vi "Periodic Tasks.vi"(8 "error in":errorcluster) -> ()   [LabVIEW 2013]
doc: "This VI runs in parallel to other tasks. It can contain as many user-defined periodic loops as you need. These can carry out PID or other sorts of timed response."
uses:
  <vilib>/Rock Robotics/SystemInterfaces/Utilities/FPGA_UtilitiesLED Source.ctl
  <vilib>/Rock Robotics/SystemInterfaces/Utilities/FPGA_UtilitiesLED State.ctl
  <vilib>/Rock Robotics/WPI/Joystick/WPI_JoystickGetSetRefNum.vi
  Robot Global Data.vi
  <vilib>/addons/control/pid/pid.llb/PID (DBL).vi
  <vilib>/addons/control/pid/NI_PID_pid.lvlib
panel:
  out "Voltage 2":dbl
  out "Voltage":dbl
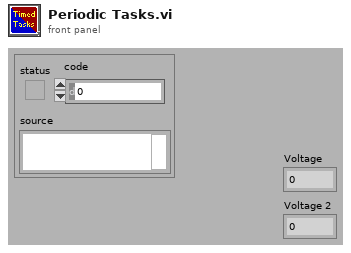
[diagram p1: front panel]
types:
  T1 = typedef "WPI_EncoderDevRef.ctl" = cluster{"DevStatus":errorcluster, "EncoderIndex":T2, "CounterIndex":T3, "DistancePerCount":dbl, "Decoding Type":T4}
  T2 = typedef "FPGA_EncoderIdx.ctl" = enum8{"Enc 0", "Enc 1", "Enc 2", "Enc 3", "Invalid"}
  T3 = typedef "FPGA_CounterCtrSystemIndex.ctl" = enum8{"Ctr 0", "Ctr 1", "Ctr 2", "Ctr 3", "Ctr 4", "Ctr 5", "Ctr 6", "Ctr 7", "Invalid"}
  T4 = typedef "WPI_EncoderType.ctl" = enum16{"1x", "2x", "4x"}
  T5 = typedef "WPI_MotorControlDeviceRef.ctl" = cluster{"DeviceStatus":errorcluster, "Type":enum16{"PWM", "CAN"}, "PWM":cluster{"Digital Module":T6, "PWM Channel":T7, "DeadBand":T8}, "CAN":cluster{"Device Number":u8, "Control Mode":T9, "Semaphore":T10, "Max Vout":dbl}, "Invert":bool, "TransformRef":T11, "InvTransformRef":T11}
  T6 = typedef "FPGA_TypedefDigitalModule.ctl" = enum16{"Digital Module 1", "Digital Module 2"}
  T7 = typedef "FPGA_DIOPWMChannel.ctl" = enum8{"PWM 1", "PWM 2", "PWM 3", "PWM 4", "PWM 5", "PWM 6", "PWM 7", "PWM 8", "PWM 9", "PWM 10", "Invalid"}
  T8 = typedef "WPI_PWMDeadband.ctl" = cluster{"Name":string, "maxPositivePwm":i32, "minPositivePwm":i32, "centerPwm":i32, "maxNegativePwm":i32, "minNegativePwm":i32, "angularRange":u16}
  T9 = typedef "WPI_CANJaguar_ControlMode.ctl" = enum8{"Percent VBus", "Current", "Speed", "Position", "Voltage"}
  T10 = typedef "Semaphore RefNum" = refnum<k1>
  T11 = typedef "WPI_PWMTransform_ConPane.ctl" = refnum<vi>
  T12 = typedef "WPI_AnalogChannelDevRef.ctl" = cluster{"DevStatus":errorcluster, "Analog Module":T13, "Analog Channel":T14}
  T13 = typedef "FPGA_TypedefAnalogModule.ctl" = enum16{"Analog Module 1", "Analog Module 2"}
  T14 = typedef "FPGA_AIChannel.ctl" = enum8{"AI 1", "AI 2", "AI 3", "AI 4", "AI 5", "AI 6", "AI 7", "AI 8", "Invalid"}
  T15 = typedef "WPI_JoystickDevRef.ctl" = cluster{"Device":T16}
  T16 = typedef "WPI_JoystickDeviceEnum.ctl" = enum16{"USB 1", "USB 2", "USB 3", "USB 4", "Kinect 1", "Kinect 2"}
  T17 = cluster{"proportional gain (Kc)":dbl, "integral time (Ti, min)":dbl, "derivative time (Td, min)":dbl}
  T18 = enum16{"Default", "Set", "Pickup", "Place", "KickerUp", "Rest", "Kick", "Rest2", "Up", "End"}
  T19 = enum16{"Default", "Set", "Pickup", "Place", "KickerUp", "Rest", "Kick", "End"}
  T20 = cluster{dbl, "integral time (Ti, min)":dbl, "derivative time (Td, min)":dbl}
  T21 = typedef "WPI_JoystickButtonState.ctl" = cluster{"Button 1":bool, "Button 2":bool, "Button 3":bool, "Button 4":bool, "Button 5":bool, "Button 6":bool, "Button 7":bool, "Button 8":bool, "Button 9":bool, "Button 10":bool, "Button 11":bool, "Button 12":bool}
  T22 = cluster{"axis 1 (x)":dbl, "axis 2 (y)":dbl, "axis 3 (throttle)":dbl, "axis 4":dbl, "axis 5":dbl, "axis 6":dbl}
  T23 = typedef "FPGA_UtilitiesLED State.ctl" = enum16{"Off", "On", "Toggle"}
  T24 = typedef "FPGA_UtilitiesLED Source.ctl" = enum16{"User LED", "FPGA LED"}
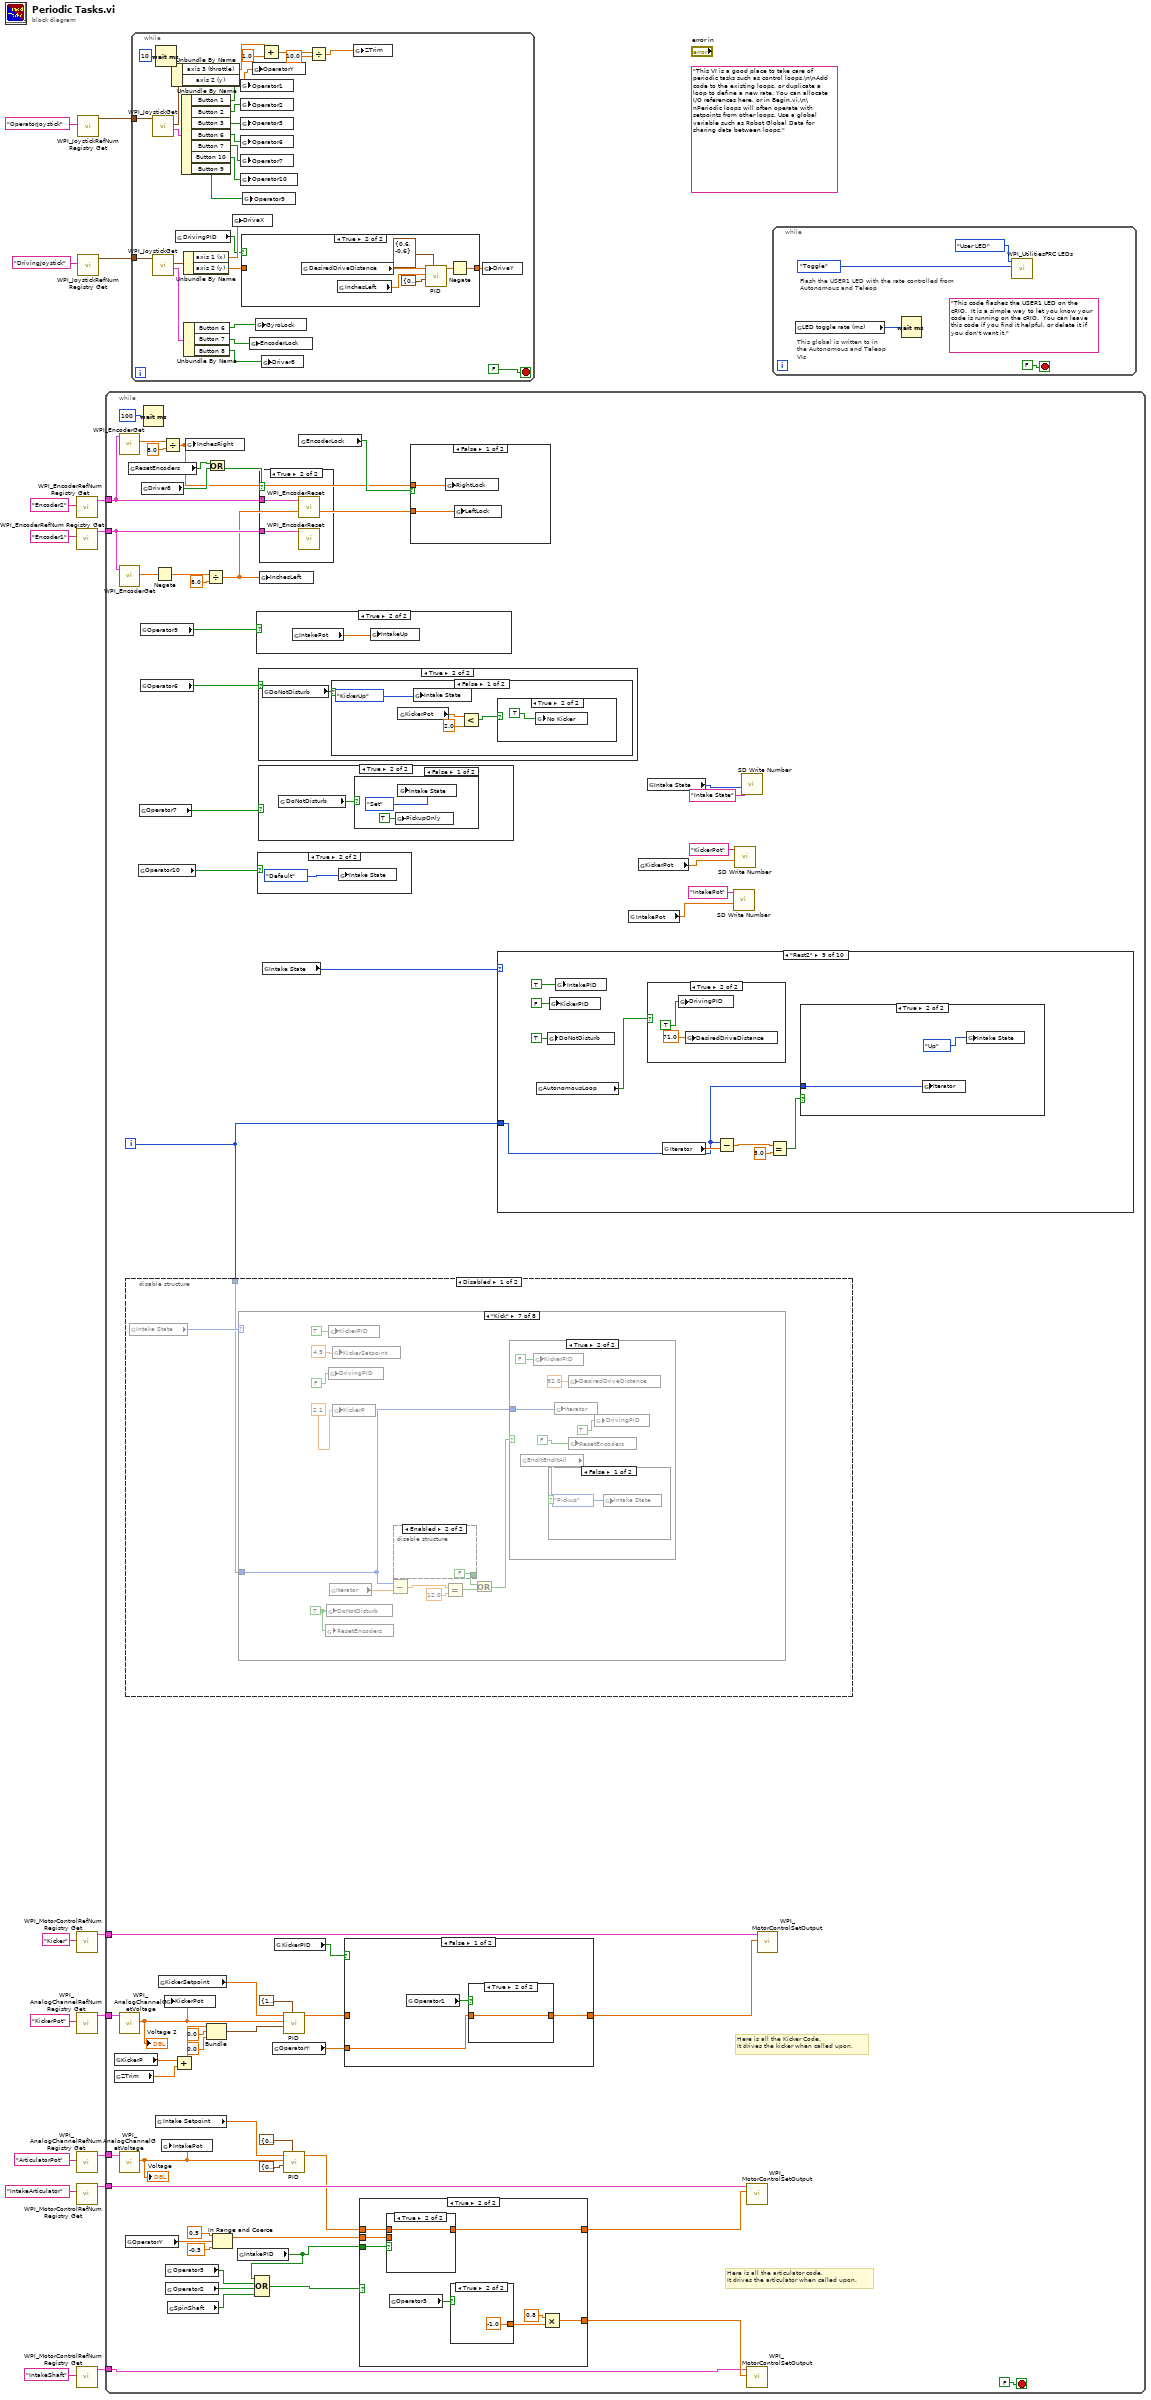
[diagram p0: block diagram]
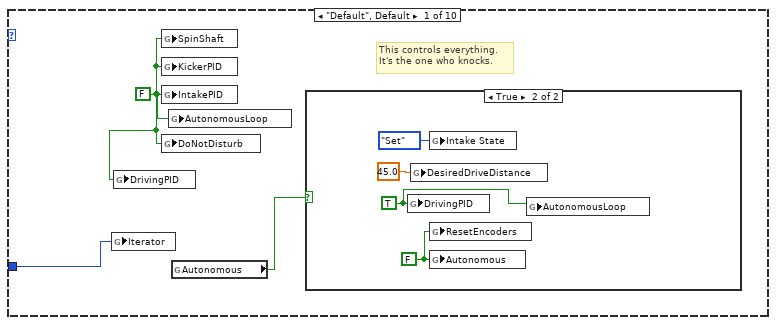
[diagram p2: hidden frame]
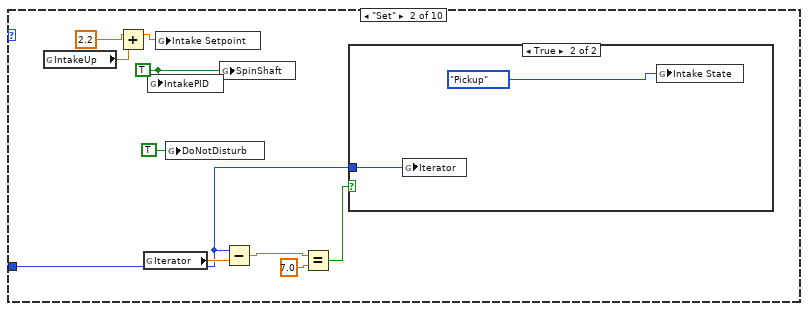
[diagram p4: hidden frame]
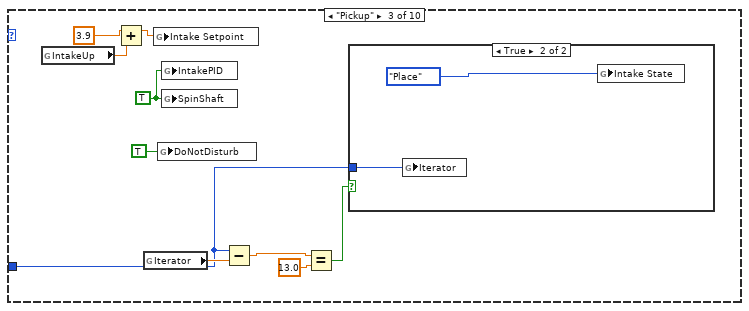
[diagram p6: hidden frame]
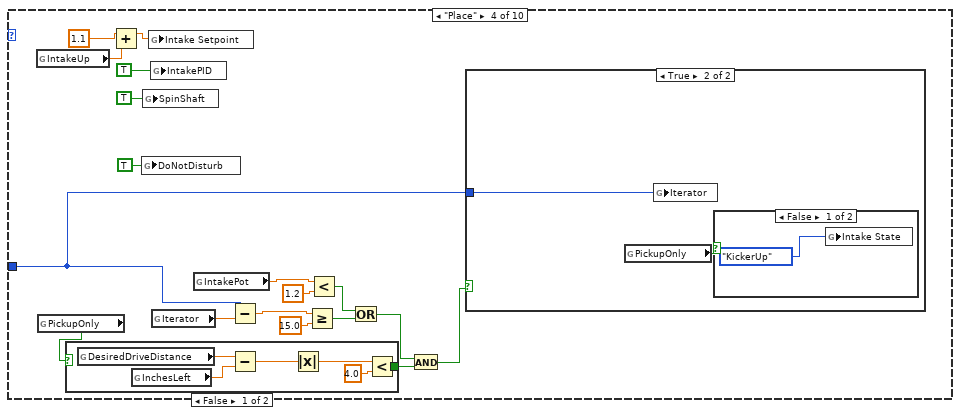
[diagram p8: hidden frame]
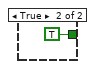
[diagram p9: hidden frame]
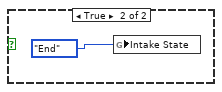
[diagram p11: hidden frame]
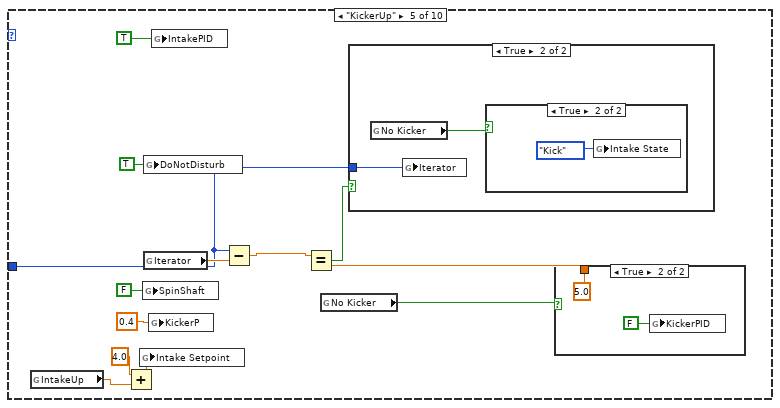
[diagram p12: hidden frame]
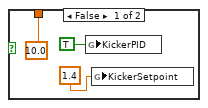
[diagram p13: hidden frame]
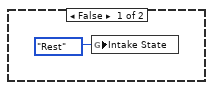
[diagram p15: hidden frame]
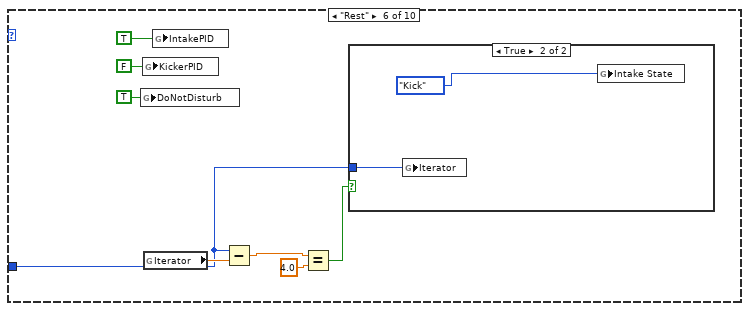
[diagram p16: hidden frame]
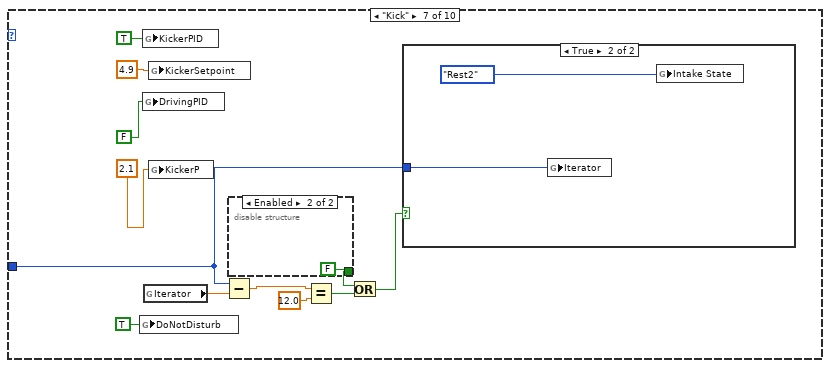
[diagram p18: hidden frame]
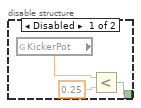
[diagram p19: hidden frame]
diagram:
  (unwired) "This VI is a good place to take care of periodic tasks such as control loops.\n\nAdd code to the existing loops, or duplicate a loop to define a new rate. You can allocate I/O references here, or in Begin.vi.\n\nPeriodic loops will often operate with setpoints from other loops. Use a global variable such as Robot Global Data for sharing data between loops."
  n1 = call <vilib>:"WPI_EncoderRefNum Registry Get.vi"("refnum name"="Encoder2") -> ("EncoderDevRef"=w12:T1)  [unwired: 9 in, 1 out]
  n2 = call <vilib>:"WPI_EncoderRefNum Registry Get.vi"("refnum name"="Encoder1") -> ("EncoderDevRef"=w13:T1)  [unwired: 9 in, 1 out]
  n3 = call <vilib>:"WPI_MotorControlRefNum Registry Get.vi"("refnum name"="Kicker") -> ("MotorControlDevRef"=w7:T5)  [unwired: 9 in, 1 out]
  n4 = call <vilib>:"WPI_AnalogChannelRefNum Registry Get.vi"("refnum name"="KickerPot") -> ("AIDeviceRef"=w4:T12)  [unwired: 9 in, 1 out]
  n5 = call <vilib>:"WPI_AnalogChannelRefNum Registry Get.vi"("refnum name"="ArticulatorPot") -> ("AIDeviceRef"=w3:T12)  [unwired: 9 in, 1 out]
  n6 = call <vilib>:"WPI_MotorControlRefNum Registry Get.vi"("refnum name"="IntakeArticulator") -> ("MotorControlDevRef"=w17:T5)  [unwired: 9 in, 1 out]
  n7 = call <vilib>:"WPI_MotorControlRefNum Registry Get.vi"("refnum name"="IntakeShaft") -> ("MotorControlDevRef"=w14:T5)  [unwired: 9 in, 1 out]
  n8 = call <vilib>:"WPI_JoystickRefNum Registry Get.vi"("refnum name"="OperatorJoystick") -> ("JoystickDevRef"=w1:T15)  [unwired: 9 in, 1 out]
  n9 = call <vilib>:"WPI_JoystickRefNum Registry Get.vi"("refnum name"="DrivingJoystick") -> ("JoystickDevRef"=w9:T15)  [unwired: 9 in, 1 out]
  n10 = while {
    tunnel: w17 -> [w77]
    tunnel: w14 -> [w75]
    tunnel: w13 -> [w59]
    tunnel: w12 -> [w62]
    tunnel: w7 -> [w70]
    tunnel: w4 -> [w69]
    tunnel: w3 -> [w68]
    i -> [w28]
    stop <- FALSE stop-if-true
    # "Here is all the articulator code. \nIt drives the articulator when called upon."
    # "Here is all the Kicker Code. \nIt drives the kicker when called upon."
    n11 = global read "Robot Global Data.vi" "KickerP"() -> (w50:dbl)
    n12 = global read "Robot Global Data.vi" "ZTrim"() -> (w32:dbl)
    n13 = call <vilib>:"WPI_EncoderGet.vi"("EncoderDevRef"=w62) -> ("Distance"=w73:dbl)  [unwired: 5 in, 5 out]
    n14 = call <vilib>:"WPI_EncoderGet.vi"("EncoderDevRef"=w59) -> ("Distance"=w74:dbl)  [unwired: 5 in, 5 out]
    n15 = call <vilib>:"WPI_AnalogChannelGetVoltage.vi"("AIDeviceRef"=w69) -> ("Voltage"=w41:dbl)  [unwired: 8 in, 2 out]
    "Voltage 2" <- w41
    n16 = call <vilib>:"WPI_AnalogChannelGetVoltage.vi"("AIDeviceRef"=w68) -> ("Voltage"=w40:dbl)  [unwired: 8 in, 2 out]
    "Voltage" <- w40
    n17 = global read "Robot Global Data.vi" "OperatorY"() -> (w46:dbl)
    n18 = disable-structure shown="Disabled" {
      disable-tunnel: w28 -> [w220 _]
      frame Disabled {
        n19 = global read "Robot Global Data.vi" "Intake State"() -> (w221:T18)
        n20 = case shown="\"Kick\"" w221 {
          tunnel: w220 -> [w224 w232 w244 w268 w285 w299 w311 _]
          frame "Default", Default {
            w222 = FALSE ("PID")
            # "This controls everything. \nIt's the one who knocks."
            n21 = global write "Robot Global Data.vi" "Iterator"(w224) -> ()
            n22 = global read "Robot Global Data.vi" "Operator7"() -> (w223:bool)
            n23 = global write "Robot Global Data.vi" "SpinShaft"(w222) -> ()
            n24 = global write "Robot Global Data.vi" "KickerPID"(w222) -> ()
            n25 = global write "Robot Global Data.vi" "IntakePID"(w222) -> ()
            n26 = global write "Robot Global Data.vi" "DoNotDisturb"(w222) -> ()
            n27 = global write "Robot Global Data.vi" "EndItEndItAll"(w222) -> ()
            n28 = case shown="True" w223 {
              frame False {
              }
              frame True {
                w225 = FALSE ("Autonomous")
                n29 = global write "Robot Global Data.vi" "Intake State"(T19."Set" ("Intake State")) -> ()
                n30 = global write "Robot Global Data.vi" "ResetEncoders"(w225) -> ()
                n31 = global write "Robot Global Data.vi" "Autonomous"(w225) -> ()
              }
            }
          }
          frame "Set" {
            w231 = TRUE ("PID")
            n32 = global read "Robot Global Data.vi" "IntakeUp"() -> (w229:dbl)
            n33 = Add(x=1.1 ("Intake Setpoint"), y=w229) -> (x+y=w228:dbl)
            n34 = global read "Robot Global Data.vi" "Iterator"() -> (w236:dbl)
            n35 = global write "Robot Global Data.vi" "IntakePID"(w231) -> ()
            n36 = global write "Robot Global Data.vi" "Intake Setpoint"(w228) -> ()
            n37 = global write "Robot Global Data.vi" "DoNotDisturb"(TRUE ("DoNotDisturb")) -> ()
            n38 = global write "Robot Global Data.vi" "SpinShaft"(w231) -> ()
            n39 = Subtract(x=w232, y=w236) -> (x-y=w235:dbl)
            n40 = Equal?(x=w235, y=9.0) -> (x = y?=w233:bool)
            n41 = case shown="True" w233 {
              tunnel: w232 -> [_ w238]
              frame False {
              }
              frame True {
                n42 = global write "Robot Global Data.vi" "Iterator"(w238) -> ()
                n43 = global write "Robot Global Data.vi" "Intake State"(T19."KickerUp" ("Intake State")) -> ()
              }
            }
          }
          frame "Pickup" {
            w243 = TRUE ("PID")
            n44 = global read "Robot Global Data.vi" "InchesRight"() -> (w240:dbl)
            n45 = global read "Robot Global Data.vi" "Iterator"() -> (w248:dbl)
            n46 = global write "Robot Global Data.vi" "DoNotDisturb"(TRUE ("DoNotDisturb")) -> ()
            n47 = Greater?(x=w240, y=24.0) -> (0:w241:bool)
            n48 = global write "Robot Global Data.vi" "IntakePID"(w243) -> ()
            n49 = global write "Robot Global Data.vi" "SpinShaft"(w243) -> ()
            n50 = case shown="False" w241 {
              frame False {
                n51 = global read "Robot Global Data.vi" "IntakeUp"() -> (w249:dbl)
                n52 = Add(x=1.1 ("Intake Setpoint"), y=w249) -> (x+y=w250:dbl)
                n53 = global write "Robot Global Data.vi" "Intake Setpoint"(w250) -> ()
              }
              frame True {
                n54 = global read "Robot Global Data.vi" "IntakeUp"() -> (w252:dbl)
                n55 = Add(x=3.9 ("Intake Setpoint"), y=w252) -> (x+y=w253:dbl)
                n56 = global write "Robot Global Data.vi" "Intake Setpoint"(w253) -> ()
              }
            }
            n57 = Subtract(x=w244, y=w248) -> (x-y=w247:dbl)
            n58 = Equal?(x=w247, y=20.0) -> (x = y?=w245:bool)
            n59 = case shown="False" w245 {
              tunnel: w244 -> [_ w256]
              frame False {
              }
              frame True {
                n60 = global write "Robot Global Data.vi" "Iterator"(w256) -> ()
                n61 = global write "Robot Global Data.vi" "Intake State"(T19."Place" ("Intake State")) -> ()
              }
            }
          }
          frame "Place" {
            w257 = TRUE ("DoNotDisturb")
            n62 = global read "Robot Global Data.vi" "IntakeUp"() -> (w260:dbl)
            n63 = global read "Robot Global Data.vi" "PickupOnly"() -> (w259:bool)
            n64 = case shown="True" w259 {
              tunnel: [w274 TRUE] -> _
              frame False {
                n65 = global read "Robot Global Data.vi" "DesiredDriveDistance"() -> (w278:dbl)
                n66 = global read "Robot Global Data.vi" "InchesRight"() -> (w273:dbl)
                n67 = Subtract(x=w278, y=w273) -> (x-y=w277:dbl)
                n68 = Absolute Value(x=w277) -> (abs(x)=w276:dbl)
                n69 = Less?(x=w276, y=2.0) -> (x < y?=w274:bool)
              }
              frame True {
              }
            }
            n70 = Add(x=1.1 ("Intake Setpoint"), y=w260) -> (x+y=w261:dbl)
            n71 = global write "Robot Global Data.vi" "EndItEndItAll"(w257) -> ()
            n72 = global write "Robot Global Data.vi" "DoNotDisturb"(w257) -> ()
            n73 = global write "Robot Global Data.vi" "SpinShaft"(TRUE ("PID")) -> ()
            n74 = global write "Robot Global Data.vi" "Intake Setpoint"(w261) -> ()
            n75 = global write "Robot Global Data.vi" "IntakePID"(TRUE ("PID")) -> ()
            n76 = global read "Robot Global Data.vi" "Iterator"() -> (w272:dbl)
            n77 = global read "Robot Global Data.vi" "IntakePot"() -> (w263:dbl)
            n78 = Subtract(x=w268, y=w272) -> (x-y=w271:dbl)
            n79 = Equal?(x=w271, y=15.0) -> (x = y?=w269:bool)
            n80 = Less?(x=w263, y=1.4) -> (x < y?=w264:bool)
            n81 = Or(x=w264, y=w269) -> (x .or. y?=w258:bool)
            n82 = case shown="True" w258 {
              tunnel: w268 -> [_ w281]
              frame False {
              }
              frame True {
                n83 = global write "Robot Global Data.vi" "Iterator"(w281) -> ()
                n84 = global write "Robot Global Data.vi" "Intake State"(T19."KickerUp" ("Intake State")) -> ()
              }
            }
          }
          frame "KickerUp" {
            n85 = global read "Robot Global Data.vi" "IntakeUp"() -> (w282:dbl)
            n86 = Add(x=4.0 ("Intake Setpoint"), y=w282) -> (x+y=w283:dbl)
            n87 = global write "Robot Global Data.vi" "Intake Setpoint"(w283) -> ()
            n88 = global write "Robot Global Data.vi" "KickerPID"(TRUE ("PID")) -> ()
            n89 = global write "Robot Global Data.vi" "SpinShaft"(FALSE ("PID")) -> ()
            n90 = global write "Robot Global Data.vi" "DoNotDisturb"(TRUE ("DoNotDisturb")) -> ()
            n91 = global read "Robot Global Data.vi" "Iterator"() -> (w289:dbl)
            n92 = global write "Robot Global Data.vi" "KickerSetpoint"(1.4 ("KickerSetpoint")) -> ()
            n93 = global write "Robot Global Data.vi" "KickerP"(0.4 ("KickerP")) -> ()
            n94 = global write "Robot Global Data.vi" "IntakePID"(TRUE ("PID")) -> ()
            n95 = Subtract(x=w285, y=w289) -> (x-y=w288:dbl)
            n96 = Equal?(x=w288, y=10.0) -> (x = y?=w286:bool)
            n97 = case shown="True" w286 {
              tunnel: w285 -> [_ w297]
              frame False {
              }
              frame True {
                n98 = global write "Robot Global Data.vi" "Iterator"(w297) -> ()
                n99 = global write "Robot Global Data.vi" "Intake State"(T19."Rest" ("Intake State")) -> ()
              }
            }
          }
          frame "Rest" {
            n100 = global write "Robot Global Data.vi" "DoNotDisturb"(TRUE ("DoNotDisturb")) -> ()
            n101 = global write "Robot Global Data.vi" "KickerPID"(FALSE ("PID")) -> ()
            n102 = global read "Robot Global Data.vi" "Iterator"() -> (w303:dbl)
            n103 = global write "Robot Global Data.vi" "IntakePID"(TRUE ("PID")) -> ()
            n104 = Subtract(x=w299, y=w303) -> (x-y=w302:dbl)
            n105 = Equal?(x=w302, y=3.0) -> (x = y?=w300:bool)
            n106 = case shown="True" w300 {
              tunnel: w299 -> [_ w307]
              frame False {
              }
              frame True {
                n107 = global write "Robot Global Data.vi" "Iterator"(w307) -> ()
                n108 = global write "Robot Global Data.vi" "Intake State"(T19."Kick" ("Intake State")) -> ()
              }
            }
          }
          frame "Kick" {
            w308 = TRUE ("DoNotDisturb")
            n109 = global write "Robot Global Data.vi" "ResetEncoders"(w308) -> ()
            n110 = global write "Robot Global Data.vi" "DoNotDisturb"(w308) -> ()
            n111 = global write "Robot Global Data.vi" "KickerPID"(TRUE ("PID")) -> ()
            n112 = global write "Robot Global Data.vi" "DrivingPID"(FALSE ("DrivingPID")) -> ()
            n113 = global read "Robot Global Data.vi" "Iterator"() -> (w314:dbl)
            n114 = global write "Robot Global Data.vi" "KickerSetpoint"(4.9 ("KickerSetpoint")) -> ()
            n115 = global write "Robot Global Data.vi" "KickerP"(2.1 ("KickerP")) -> ()
            n116 = Subtract(x=w311, y=w314) -> (x-y=w313:dbl)
            n117 = disable-structure shown="Enabled" {
              disable-tunnel: [w321 FALSE] -> w316
              frame Disabled {
                n118 = global read "Robot Global Data.vi" "KickerPot"() -> (w320:dbl)
                n119 = Less?(x=w320, y=0.25) -> (x < y?=w321:bool)
              }
              frame Enabled {
              }
            }
            n120 = Equal?(x=w313, y=12.0) -> (x = y?=w309:bool)
            n121 = Or(x=w316, y=w309) -> (x .or. y?=w310:bool)
            n122 = case shown="True" w310 {
              tunnel: w311 -> [_ w329]
              frame False {
              }
              frame True {
                n123 = global read "Robot Global Data.vi" "EndItEndItAll"() -> (w325:bool)
                n124 = global write "Robot Global Data.vi" "KickerPID"(FALSE ("PID")) -> ()
                n125 = case shown="False" w325 {
                  frame False {
                    n126 = global write "Robot Global Data.vi" "Intake State"(T19."Pickup" ("Intake State")) -> ()
                  }
                  frame True {
                    n127 = global write "Robot Global Data.vi" "Intake State"(T19."End" ("Intake State")) -> ()
                  }
                }
                n128 = global write "Robot Global Data.vi" "Iterator"(w329) -> ()
                n129 = global write "Robot Global Data.vi" "DesiredDriveDistance"(92.0 ("DesiredDriveDistance")) -> ()
                n130 = global write "Robot Global Data.vi" "ResetEncoders"(FALSE ("DrivingPID")) -> ()
                n131 = global write "Robot Global Data.vi" "DrivingPID"(TRUE ("DrivingPID")) -> ()
              }
            }
          }
          frame "End" {
            w332 = FALSE ("DoNotDisturb")
            w333 = FALSE ("PID")
            n132 = global write "Robot Global Data.vi" "DoNotDisturb"(w332) -> ()
            n133 = global write "Robot Global Data.vi" "KickerPID"(FALSE ("PID")) -> ()
            n134 = global write "Robot Global Data.vi" "IntakePID"(w333) -> ()
            n135 = global write "Robot Global Data.vi" "DrivingPID"(w333) -> ()
            n136 = global write "Robot Global Data.vi" "Intake State"(T19."Default" ("Intake State")) -> ()
            n137 = global write "Robot Global Data.vi" "PickupOnly"(w332) -> ()
          }
        }
      }
      frame Enabled {
      }
    }
    n138 = global read "Robot Global Data.vi" "ResetEncoders"() -> (w35:bool)
    n139 = global read "Robot Global Data.vi" "Operator10"() -> (w37:bool)
    n140 = global read "Robot Global Data.vi" "Operator7"() -> (w38:bool)
    n141 = global read "Robot Global Data.vi" "Operator9"() -> (w31:bool)
    n142 = global read "Robot Global Data.vi" "Operator6"() -> (w39:bool)
    n143 = global read "Robot Global Data.vi" "Driver8"() -> (w34:bool)
    n144 = Wait (ms)(milliseconds to wait=u32 100) -> ()  [unwired: 1 out]
    n145 = Negate(x=w74) -> (-x=w58:dbl)
    n146 = global read "Robot Global Data.vi" "Intake Setpoint"() -> (w63:dbl)
    n147 = global read "Robot Global Data.vi" "KickerSetpoint"() -> (w49:dbl)
    n148 = global write "Robot Global Data.vi" "IntakePot"(w40) -> ()
    n149 = Divide(x=w73, y=8.0) -> (x/y=w19:dbl)
    n150 = global write "Robot Global Data.vi" "KickerPot"(w41) -> ()
    n151 = global read "Robot Global Data.vi" "Operator3"() -> (w43:bool)
    n152 = global read "Robot Global Data.vi" "Operator2"() -> (w42:bool)
    n153 = global read "Robot Global Data.vi" "SpinShaft"() -> (w54:bool)
    n154 = Add(x=w50, y=w32) -> (x+y=w33:dbl)
    n155 = global write "Robot Global Data.vi" "InchesRight"(w19) -> ()
    n156 = Divide(x=w58, y=8.0) -> (x/y=w20:dbl)
    n157 = Bundle(w33, "integral time (Ti, min)"=0.0, "derivative time (Td, min)"=0.0) -> (w53:T20)  [unwired: 1 in]
    n158 = Or(x=w35, y=w34) -> (x .or. y?=w36:bool)
    n159 = In Range and Coerce(upper limit=0.5, x=w46, lower limit=-0.5) -> (coerced(x)=w60:dbl)  [unwired: 1 out]
    n160 = global read "Robot Global Data.vi" "IntakePID"() -> (w30:bool)
    n161 = Compound Arithmetic op=OR(w30, w43, w42, w54) -> (w72:bool)
    n162 = case shown="True" w31 {
      frame False {
      }
      frame True {
        n163 = global read "Robot Global Data.vi" "IntakePot"() -> (w338:dbl)
        n164 = global write "Robot Global Data.vi" "IntakeUp"(w338) -> ()
      }
    }
    n165 = case shown="True" w37 {
      frame False {
      }
      frame True {
        n166 = global write "Robot Global Data.vi" "Intake State"(T18."Default" ("Intake State")) -> ()
      }
    }
    n167 = case shown="True" w39 {
      frame False {
      }
      frame True {
        n168 = global read "Robot Global Data.vi" "DoNotDisturb"() -> (w343:bool)
        n169 = case shown="False" w343 {
          frame False {
            n170 = global read "Robot Global Data.vi" "KickerPot"() -> (w346:dbl)
            n171 = global write "Robot Global Data.vi" "Intake State"(T18."KickerUp" ("Intake State")) -> ()
            n172 = Less?(x=w346, y=2.0) -> (x < y?=w344:bool)
            n173 = case shown="True" w344 {
              frame False {
                n174 = global write "Robot Global Data.vi" "No Kicker"(FALSE) -> ()
              }
              frame True {
                n175 = global write "Robot Global Data.vi" "No Kicker"(TRUE) -> ()
              }
            }
          }
          frame True {
          }
        }
      }
    }
    n176 = case shown="True" w38 {
      frame False {
      }
      frame True {
        n177 = global read "Robot Global Data.vi" "DoNotDisturb"() -> (w340:bool)
        n178 = case shown="False" w340 {
          frame False {
            n179 = global write "Robot Global Data.vi" "PickupOnly"(TRUE ("PickupOnly")) -> ()
            n180 = global write "Robot Global Data.vi" "Intake State"(T18."Set" ("Intake State")) -> ()
          }
          frame True {
          }
        }
      }
    }
    n181 = case shown="True" w36 {
      tunnel: w62 -> [_ w351]
      tunnel: w59 -> [_ w350]
      frame False {
      }
      frame True {
        n182 = call <vilib>:"WPI_EncoderReset.vi"("EncoderDevRef"=w351) -> ()  [unwired: 9 in, 2 out]
        n183 = call <vilib>:"WPI_EncoderReset.vi"("EncoderDevRef"=w350) -> ()  [unwired: 9 in, 2 out]
      }
    }
    n184 = global write "Robot Global Data.vi" "InchesLeft"(w20) -> ()
    n185 = global read "Robot Global Data.vi" "Intake State"() -> (w27:T18)
    n186 = global read "Robot Global Data.vi" "OperatorY"() -> (w47:dbl)
    n187 = global read "Robot Global Data.vi" "KickerPID"() -> (w48:bool)
    n188 = call-poly <vilib>:"PID.vi"("output range"=cluster{"output high":dbl, "output low":dbl} {"output high"=1.0, "output low"=-0.9}, "PID gains"=w53, "process variable"=w41, "setpoint"=w49) -> ("output"=w64:dbl)  [unwired: 6 in, 1 out]
    n189 = call-poly <vilib>:"PID.vi"("output range"=cluster{"output high":dbl, "output low":dbl} {"output high"=0.7, "output low"=-0.7}, "PID gains"=T17 {"proportional gain (Kc)"=0.4, "integral time (Ti, min)"=0.0, "derivative time (Td, min)"=0.0}, "process variable"=w40, "setpoint"=w63) -> ("output"=w55:dbl)  [unwired: 6 in, 1 out]
    n190 = global read "Robot Global Data.vi" "EncoderLock"() -> (w29:bool)
    n191 = case shown="False" w48 {
      tunnel: [w354 w357] -> w71
      tunnel: w64 -> [_ w357]
      tunnel: w47 -> [w353 _]
      frame False {
        n192 = global read "Robot Global Data.vi" "Operator1"() -> (w352:bool)
        n193 = case shown="True" w352 {
          tunnel: [0 w356] -> w354
          tunnel: w353 -> [_ w356]
          frame False {
          }
          frame True {
          }
        }
      }
      frame True {
      }
    }
    n194 = case shown="True" w72 {
      tunnel: [0 w366] -> w76
      tunnel: [0.0 ("output") w363] -> w61
      tunnel: w60 -> [_ w362]
      tunnel: w55 -> [_ w361]
      tunnel: w30 -> [_ w364]
      frame False {
      }
      frame True {
        n195 = case shown="True" w364 {
          tunnel: [w368 w369] -> w363
          tunnel: w362 -> [w368 _]
          tunnel: w361 -> [_ w369]
          frame False {
          }
          frame True {
          }
        }
        n196 = global read "Robot Global Data.vi" "Operator3"() -> (w360:bool)
        n197 = case shown="True" w360 {
          tunnel: [1.0 ("y") -1.0 ("y")] -> w365
          frame False {
          }
          frame True {
          }
        }
        n198 = Multiply(x=0.8 ("ShaftSpeed"), y=w365) -> (x*y=w366:dbl)
      }
    }
    n199 = case shown="False" w29 {
      tunnel: w19 -> [w337 _]
      tunnel: w20 -> [w336 _]
      frame False {
        n200 = global write "Robot Global Data.vi" "RightLock"(w337) -> ()
        n201 = global write "Robot Global Data.vi" "LeftLock"(w336) -> ()
      }
      frame True {
      }
    }
    n202 = case shown="\"Rest2\"" w27 {
      tunnel: w28 -> [w82 w92 w104 w124 w145 w163 w175 _ w195 w207]
      frame "Default", Default {
        w80 = FALSE ("PID")
        # "This controls everything. \nIt's the one who knocks."
        n203 = global write "Robot Global Data.vi" "Iterator"(w82) -> ()
        n204 = global write "Robot Global Data.vi" "DrivingPID"(w80) -> ()
        n205 = global write "Robot Global Data.vi" "SpinShaft"(w80) -> ()
        n206 = global write "Robot Global Data.vi" "KickerPID"(w80) -> ()
        n207 = global write "Robot Global Data.vi" "IntakePID"(w80) -> ()
        n208 = global write "Robot Global Data.vi" "DoNotDisturb"(w80) -> ()
        n209 = global write "Robot Global Data.vi" "AutonomousLoop"(w80) -> ()
        n210 = global read "Robot Global Data.vi" "Autonomous"() -> (w81:bool)
        n211 = case shown="True" w81 {
          frame False {
          }
          frame True {
            w83 = TRUE ("PID")
            w85 = FALSE ("Autonomous")
            n212 = global write "Robot Global Data.vi" "DrivingPID"(w83) -> ()
            n213 = global write "Robot Global Data.vi" "DesiredDriveDistance"(45.0 ("DesiredDriveDistance")) -> ()
            n214 = global write "Robot Global Data.vi" "Intake State"(T18."Set" ("Intake State")) -> ()
            n215 = global write "Robot Global Data.vi" "ResetEncoders"(w85) -> ()
            n216 = global write "Robot Global Data.vi" "Autonomous"(w85) -> ()
            n217 = global write "Robot Global Data.vi" "AutonomousLoop"(w83) -> ()
          }
        }
      }
      frame "Set" {
        w91 = TRUE ("PID")
        n218 = global read "Robot Global Data.vi" "IntakeUp"() -> (w89:dbl)
        n219 = Add(x=2.2 ("Intake Setpoint"), y=w89) -> (x+y=w88:dbl)
        n220 = global read "Robot Global Data.vi" "Iterator"() -> (w96:dbl)
        n221 = global write "Robot Global Data.vi" "IntakePID"(w91) -> ()
        n222 = global write "Robot Global Data.vi" "Intake Setpoint"(w88) -> ()
        n223 = global write "Robot Global Data.vi" "DoNotDisturb"(TRUE ("DoNotDisturb")) -> ()
        n224 = global write "Robot Global Data.vi" "SpinShaft"(w91) -> ()
        n225 = Subtract(x=w92, y=w96) -> (x-y=w95:dbl)
        n226 = Equal?(x=w95, y=7.0) -> (x = y?=w93:bool)
        n227 = case shown="True" w93 {
          tunnel: w92 -> [_ w98]
          frame False {
          }
          frame True {
            n228 = global write "Robot Global Data.vi" "Iterator"(w98) -> ()
            n229 = global write "Robot Global Data.vi" "Intake State"(T18."Pickup" ("Intake State")) -> ()
          }
        }
      }
      frame "Pickup" {
        w103 = TRUE ("PID")
        n230 = global read "Robot Global Data.vi" "IntakeUp"() -> (w99:dbl)
        n231 = Add(x=3.9 ("Intake Setpoint"), y=w99) -> (x+y=w100:dbl)
        n232 = global read "Robot Global Data.vi" "Iterator"() -> (w108:dbl)
        n233 = global write "Robot Global Data.vi" "Intake Setpoint"(w100) -> ()
        n234 = global write "Robot Global Data.vi" "DoNotDisturb"(TRUE ("DoNotDisturb")) -> ()
        n235 = global write "Robot Global Data.vi" "IntakePID"(w103) -> ()
        n236 = global write "Robot Global Data.vi" "SpinShaft"(w103) -> ()
        n237 = Subtract(x=w104, y=w108) -> (x-y=w107:dbl)
        n238 = Equal?(x=w107, y=13.0) -> (x = y?=w105:bool)
        n239 = case shown="True" w105 {
          tunnel: w104 -> [_ w110]
          frame False {
          }
          frame True {
            n240 = global write "Robot Global Data.vi" "Iterator"(w110) -> ()
            n241 = global write "Robot Global Data.vi" "Intake State"(T18."Place" ("Intake State")) -> ()
          }
        }
      }
      frame "Place" {
        n242 = global read "Robot Global Data.vi" "IntakeUp"() -> (w112:dbl)
        n243 = global read "Robot Global Data.vi" "PickupOnly"() -> (w111:bool)
        n244 = case shown="False" w111 {
          tunnel: [w130 TRUE] -> w117
          frame False {
            n245 = global read "Robot Global Data.vi" "DesiredDriveDistance"() -> (w134:dbl)
            n246 = global read "Robot Global Data.vi" "InchesLeft"() -> (w129:dbl)
            n247 = Subtract(x=w134, y=w129) -> (x-y=w133:dbl)
            n248 = Absolute Value(x=w133) -> (abs(x)=w132:dbl)
            n249 = Less?(x=w132, y=4.0) -> (x < y?=w130:bool)
          }
          frame True {
          }
        }
        n250 = Add(x=1.1 ("Intake Setpoint"), y=w112) -> (x+y=w113:dbl)
        n251 = global write "Robot Global Data.vi" "DoNotDisturb"(TRUE ("DoNotDisturb")) -> ()
        n252 = global write "Robot Global Data.vi" "SpinShaft"(TRUE ("PID")) -> ()
        n253 = global write "Robot Global Data.vi" "Intake Setpoint"(w113) -> ()
        n254 = global write "Robot Global Data.vi" "IntakePID"(TRUE ("PID")) -> ()
        n255 = global read "Robot Global Data.vi" "Iterator"() -> (w128:dbl)
        n256 = global read "Robot Global Data.vi" "IntakePot"() -> (w116:dbl)
        n257 = Subtract(x=w124, y=w128) -> (x-y=w127:dbl)
        n258 = Greater Or Equal?(x=w127, y=15.0) -> (x >= y?=w125:bool)
        n259 = Less?(x=w116, y=1.2) -> (x < y?=w119:bool)
        n260 = Or(x=w119, y=w125) -> (x .or. y?=w121:bool)
        n261 = And(x=w121, y=w117) -> (x .and. y?=w118:bool)
        n262 = case shown="True" w118 {
          tunnel: w124 -> [_ w137]
          frame False {
          }
          frame True {
            n263 = global read "Robot Global Data.vi" "PickupOnly"() -> (w136:bool)
            n264 = global write "Robot Global Data.vi" "Iterator"(w137) -> ()
            n265 = case shown="False" w136 {
              frame False {
                n266 = global write "Robot Global Data.vi" "Intake State"(T18."KickerUp" ("Intake State")) -> ()
              }
              frame True {
                n267 = global write "Robot Global Data.vi" "Intake State"(T18."End" ("Intake State")) -> ()
              }
            }
          }
        }
      }
      frame "KickerUp" {
        n268 = global read "Robot Global Data.vi" "IntakeUp"() -> (w142:dbl)
        n269 = Add(x=4.0 ("Intake Setpoint"), y=w142) -> (x+y=w143:dbl)
        n270 = global write "Robot Global Data.vi" "Intake Setpoint"(w143) -> ()
        n271 = global write "Robot Global Data.vi" "SpinShaft"(FALSE ("PID")) -> ()
        n272 = global write "Robot Global Data.vi" "DoNotDisturb"(TRUE ("DoNotDisturb")) -> ()
        n273 = global read "Robot Global Data.vi" "Iterator"() -> (w148:dbl)
        n274 = global write "Robot Global Data.vi" "KickerP"(0.4 ("KickerP")) -> ()
        n275 = global write "Robot Global Data.vi" "IntakePID"(TRUE ("PID")) -> ()
        n276 = Subtract(x=w145, y=w148) -> (x-y=w147:dbl)
        n277 = global read "Robot Global Data.vi" "No Kicker"() -> (w140:bool)
        n278 = case shown="True" w140 {
          tunnel: [10.0 ("y") 5.0 ("y")] -> w141
          frame False {
            n279 = global write "Robot Global Data.vi" "KickerPID"(TRUE ("PID")) -> ()
            n280 = global write "Robot Global Data.vi" "KickerSetpoint"(1.4 ("KickerSetpoint")) -> ()
          }
          frame True {
            n281 = global write "Robot Global Data.vi" "KickerPID"(FALSE ("PID")) -> ()
          }
        }
        n282 = Equal?(x=w147, y=w141) -> (x = y?=w146:bool)
        n283 = case shown="True" w146 {
          tunnel: w145 -> [_ w159]
          frame False {
          }
          frame True {
            n284 = global read "Robot Global Data.vi" "No Kicker"() -> (w158:bool)
            n285 = global write "Robot Global Data.vi" "Iterator"(w159) -> ()
            n286 = case shown="True" w158 {
              frame False {
                n287 = global write "Robot Global Data.vi" "Intake State"(T18."Rest" ("Intake State")) -> ()
              }
              frame True {
                n288 = global write "Robot Global Data.vi" "Intake State"(T18."Kick" ("Intake State")) -> ()
              }
            }
          }
        }
      }
      frame "Rest" {
        n289 = global write "Robot Global Data.vi" "DoNotDisturb"(TRUE ("DoNotDisturb")) -> ()
        n290 = global write "Robot Global Data.vi" "KickerPID"(FALSE ("PID")) -> ()
        n291 = global read "Robot Global Data.vi" "Iterator"() -> (w167:dbl)
        n292 = global write "Robot Global Data.vi" "IntakePID"(TRUE ("PID")) -> ()
        n293 = Subtract(x=w163, y=w167) -> (x-y=w166:dbl)
        n294 = Equal?(x=w166, y=4.0) -> (x = y?=w164:bool)
        n295 = case shown="True" w164 {
          tunnel: w163 -> [_ w171]
          frame False {
          }
          frame True {
            n296 = global write "Robot Global Data.vi" "Iterator"(w171) -> ()
            n297 = global write "Robot Global Data.vi" "Intake State"(T18."Kick" ("Intake State")) -> ()
          }
        }
      }
      frame "Kick" {
        n298 = global write "Robot Global Data.vi" "DoNotDisturb"(TRUE ("DoNotDisturb")) -> ()
        n299 = global write "Robot Global Data.vi" "KickerPID"(TRUE ("PID")) -> ()
        n300 = global write "Robot Global Data.vi" "DrivingPID"(FALSE ("DrivingPID")) -> ()
        n301 = global read "Robot Global Data.vi" "Iterator"() -> (w178:dbl)
        n302 = global write "Robot Global Data.vi" "KickerSetpoint"(4.9 ("KickerSetpoint")) -> ()
        n303 = global write "Robot Global Data.vi" "KickerP"(2.1 ("KickerP")) -> ()
        n304 = Subtract(x=w175, y=w178) -> (x-y=w177:dbl)
        n305 = disable-structure shown="Enabled" {
          disable-tunnel: [w185 FALSE] -> w180
          frame Disabled {
            n306 = global read "Robot Global Data.vi" "KickerPot"() -> (w184:dbl)
            n307 = Less?(x=w184, y=0.25) -> (x < y?=w185:bool)
          }
          frame Enabled {
          }
        }
        n308 = Equal?(x=w177, y=12.0) -> (x = y?=w173:bool)
        n309 = Or(x=w180, y=w173) -> (x .or. y?=w174:bool)
        n310 = case shown="True" w174 {
          tunnel: w175 -> [_ w189]
          frame False {
          }
          frame True {
            n311 = global write "Robot Global Data.vi" "Iterator"(w189) -> ()
            n312 = global write "Robot Global Data.vi" "Intake State"(T18."Rest2" ("Intake State")) -> ()
          }
        }
      }
      frame "End" {
        w191 = FALSE ("DoNotDisturb")
        w193 = FALSE ("PID")
        w190 = FALSE ("PID")
        n313 = global write "Robot Global Data.vi" "DoNotDisturb"(w191) -> ()
        n314 = global write "Robot Global Data.vi" "KickerPID"(w190) -> ()
        n315 = global write "Robot Global Data.vi" "IntakePID"(w193) -> ()
        n316 = global write "Robot Global Data.vi" "DrivingPID"(w193) -> ()
        n317 = global write "Robot Global Data.vi" "SpinShaft"(w191) -> ()
        n318 = global write "Robot Global Data.vi" "Intake State"(T18."Default" ("Intake State")) -> ()
        n319 = global write "Robot Global Data.vi" "No Kicker"(w190) -> ()
        n320 = global write "Robot Global Data.vi" "PickupOnly"(w191) -> ()
      }
      frame "Rest2" {
        n321 = global read "Robot Global Data.vi" "AutonomousLoop"() -> (w194:bool)
        n322 = global write "Robot Global Data.vi" "DoNotDisturb"(TRUE ("DoNotDisturb")) -> ()
        n323 = global write "Robot Global Data.vi" "KickerPID"(FALSE ("PID")) -> ()
        n324 = global write "Robot Global Data.vi" "IntakePID"(TRUE ("PID")) -> ()
        n325 = case shown="True" w194 {
          frame False {
          }
          frame True {
            n326 = global write "Robot Global Data.vi" "DrivingPID"(TRUE ("DrivingPID")) -> ()
            n327 = global write "Robot Global Data.vi" "DesiredDriveDistance"(71.0 ("DesiredDriveDistance")) -> ()
          }
        }
        n328 = global read "Robot Global Data.vi" "Iterator"() -> (w200:dbl)
        n329 = Subtract(x=w195, y=w200) -> (x-y=w199:dbl)
        n330 = Equal?(x=w199, y=5.0) -> (x = y?=w197:bool)
        n331 = case shown="True" w197 {
          tunnel: w195 -> [_ w206]
          frame False {
          }
          frame True {
            n332 = global write "Robot Global Data.vi" "Iterator"(w206) -> ()
            n333 = global write "Robot Global Data.vi" "Intake State"(T18."Up" ("Intake State")) -> ()
          }
        }
      }
      frame "Up" {
        n334 = global read "Robot Global Data.vi" "IntakeUp"() -> (w212:dbl)
        n335 = Add(x=0.0 ("Intake Setpoint"), y=w212) -> (x+y=w213:dbl)
        n336 = global write "Robot Global Data.vi" "DoNotDisturb"(TRUE ("DoNotDisturb")) -> ()
        n337 = global write "Robot Global Data.vi" "SpinShaft"(TRUE ("PID")) -> ()
        n338 = global write "Robot Global Data.vi" "Intake Setpoint"(w213) -> ()
        n339 = global write "Robot Global Data.vi" "IntakePID"(TRUE ("PID")) -> ()
        n340 = global read "Robot Global Data.vi" "Iterator"() -> (w211:dbl)
        n341 = Subtract(x=w207, y=w211) -> (x-y=w210:dbl)
        n342 = Equal?(x=w210, y=5.0) -> (x = y?=w208:bool)
        n343 = case shown="True" w208 {
          tunnel: w207 -> [_ w219]
          frame False {
          }
          frame True {
            n344 = global write "Robot Global Data.vi" "Iterator"(w219) -> ()
            n345 = global write "Robot Global Data.vi" "Intake State"(T18."End" ("Intake State")) -> ()
          }
        }
      }
    }
    n346 = global read "Robot Global Data.vi" "IntakePot"() -> (w23:dbl)
    n347 = global read "Robot Global Data.vi" "KickerPot"() -> (w24:dbl)
    n348 = global read "Robot Global Data.vi" "Intake State"() -> (w22:T18)
    n349 = call <vilib>:"SD Write Number.vi"("Numeric"=w23, "Name"="IntakePot") -> ()  [unwired: 8 in, 2 out]
    n350 = call <vilib>:"SD Write Number.vi"("Numeric"=w24, "Name"="KickerPot") -> ()  [unwired: 8 in, 2 out]
    n351 = call <vilib>:"SD Write Number.vi"("Numeric"=w22, "Name"="Intake State") -> ()  [unwired: 8 in, 2 out]
    n352 = call <vilib>:"WPI_MotorControlSetOutput.vi"("Output"=w61, "MotorControlDevRef"=w77) -> ()  [unwired: 7 in, 3 out]
    n353 = call <vilib>:"WPI_MotorControlSetOutput.vi"("Output"=w76, "MotorControlDevRef"=w75) -> ()  [unwired: 7 in, 3 out]
    n354 = call <vilib>:"WPI_MotorControlSetOutput.vi"("Output"=w71, "MotorControlDevRef"=w70) -> ()  [unwired: 7 in, 3 out]
  }
  n355 = while {
    tunnel: w9 -> [w397]
    tunnel: w1 -> [w391]
    stop <- FALSE stop-if-true
    n356 = call <vilib>:"WPI_JoystickGet.vi"("JoystickDevRef"=w391) -> ("Buttons"=w389:T21, "Axes"=w390:T22)  [unwired: 4 in, 1 out]
    n357 = call <vilib>:"WPI_JoystickGet.vi"("JoystickDevRef"=w397) -> ("Buttons"=w381:T21, "Axes"=w396:T22)  [unwired: 4 in, 1 out]
    n358 = Wait (ms)(milliseconds to wait=u32 10) -> ()  [unwired: 1 out]
    n359 = Unbundle By Name(w390) -> ("axis 3 (throttle)"=w377:dbl, "axis 2 (y)"=w382:dbl)
    n360 = global read "Robot Global Data.vi" "DrivingPID"() -> (w392:bool)
    n361 = Unbundle By Name(w389) -> ("Button 1"=w388:bool, "Button 2"=w387:bool, "Button 3"=w386:bool, "Button 6"=w385:bool, "Button 7"=w384:bool, "Button 10"=w383:bool, "Button 9"=w372:bool)
    n362 = Unbundle By Name(w396) -> ("axis 1 (x)"=w395:dbl, "axis 2 (y)"=w394:dbl)
    n363 = Unbundle By Name(w381) -> ("Button 6"=w380:bool, "Button 7"=w379:bool, "Button 8"=w378:bool)
    n364 = global write "Robot Global Data.vi" "DriveX"(w395) -> ()
    n365 = global write "Robot Global Data.vi" "Operator1"(w388) -> ()
    n366 = global write "Robot Global Data.vi" "Operator2"(w387) -> ()
    n367 = global write "Robot Global Data.vi" "Operator3"(w386) -> ()
    n368 = global write "Robot Global Data.vi" "Operator6"(w385) -> ()
    n369 = global write "Robot Global Data.vi" "Operator7"(w384) -> ()
    n370 = global write "Robot Global Data.vi" "Operator10"(w383) -> ()
    n371 = case shown="True" w392 {
      tunnel: w394 -> [w400 _]
      tunnel: [w400 w403] -> w393
      frame False {
      }
      frame True {
        n372 = global read "Robot Global Data.vi" "DesiredDriveDistance"() -> (w401:dbl)
        n373 = global read "Robot Global Data.vi" "InchesLeft"() -> (w402:dbl)
        n374 = call-poly <vilib>:"PID.vi"("output range"=cluster{"output high":dbl, "output low":dbl} {"output high"=0.6, "output low"=-0.6}, "PID gains"=T17 {"proportional gain (Kc)"=0.085, "integral time (Ti, min)"=0.0, "derivative time (Td, min)"=0.0} ("PID gains 3"), "process variable"=w402, "setpoint"=w401) -> ("output"=w404:dbl)  [unwired: 6 in, 1 out]
        n375 = Negate(x=w404) -> (-x=w403:dbl)
      }
    }
    n376 = global write "Robot Global Data.vi" "Operator9"(w372) -> ()
    n377 = global write "Robot Global Data.vi" "EncoderLock"(w379) -> ()
    n378 = global write "Robot Global Data.vi" "OperatorY"(w382) -> ()
    n379 = global write "Robot Global Data.vi" "GyroLock"(w380) -> ()
    n380 = Add(x=w377, y=1.0) -> (x+y=w375:dbl)
    n381 = global write "Robot Global Data.vi" "Driver8"(w378) -> ()
    n382 = Divide(x=w375, y=10.0) -> (x/y=w373:dbl)
    n383 = global write "Robot Global Data.vi" "ZTrim"(w373) -> ()
    n384 = global write "Robot Global Data.vi" "DriveY"(w393) -> ()
  }
  n385 = while {
    stop <- FALSE stop-if-true
    (unwired) "This code flashes the USER1 LED on the cRIO.  It is a simple way to let you know your code is running on the cRIO.  You can leave this code if you find it helpful, or delete it if you don't want it."
    # "This global is written to in the Autonomous and Teleop VIs"
    # "Flash the USER1 LED with the rate controlled from Autonomous and Teleop"
    n386 = global read "Robot Global Data.vi" "LED toggle rate (ms)"() -> (w407:u32)
    n387 = Wait (ms)(milliseconds to wait=w407) -> ()  [unwired: 1 out]
    n388 = call <vilib>:"WPI_UtilitiesFRC LEDs.vi"("State"=FPGA_UtilitiesLED_State."Toggle", "LED Type"=FPGA_UtilitiesLED_Source."User LED") -> ()  [unwired: 1 in, 9 out]
  }
